vi "CFTS-Add Log Entry.vi"(0 "State":T1, 7 "message":string, 11 "error in (no error)":errorcluster) -> (4 "State thru":T1, 15 "error out":errorcluster)   [LabVIEW 2020]
uses:
  CFTS-Experiment State.ctl
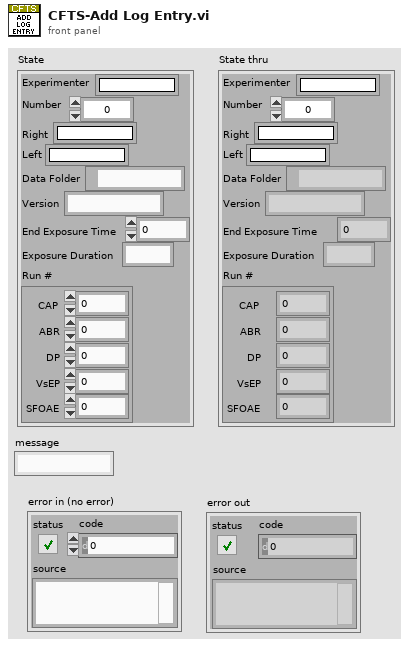
[diagram p1: front panel]
types:
  T1 = typedef "CFTS-Experiment State.ctl" = cluster{"Experimenter":string, "Number":u32, "Right":string, "Left":string, "Data Folder":path, "Version":string, "End Exposure Time":dbl, "Exposure Duration":string, "Run #":cluster{"CAP":i32, "ABR":i32, "DP":i32, "VsEP":i32, "SFOAE":i32}}
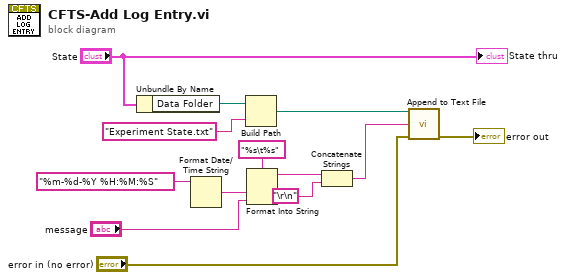
[diagram p0: block diagram]
diagram:
  n1 = Unbundle By Name("State") -> ("Data Folder"=w11:path)
  n2 = Format Date/Time String(time format string (%c)="%m-%d-%Y %H:%M:%S") -> (date/time string=w5:string)  [unwired: 2 in]
  n3 = Build Path(base path=w11, name or relative path="Experiment State.txt" ("subkey")) -> (appended path=w10:path)
  n4 = Format Into String(format string="%s\t%s", w5, "message") -> (resulting string=w4:string)  [unwired: 2 in, 1 out]
  n5 = Concatenate Strings(w4, "\r\n") -> (w2:string)
  n6 = call "Append to Text File.vi"("file path"=w10, "text"=w2, "error in (no error)"="error in (no error)") -> ("error out"=→"error out":errorcluster)  [unwired: 11 in, 1 out]
  "State thru" <- "State"
